vi "配置文件-查找多个键.vi"(6 "默认值":string[](array[string]), 8 "错误输入（无错误）":errorcluster, 9 "键名":string[](array[string]), 10 "章名":string, 11 "引用句柄输入":T1 caption="refnum") -> (0 "错误输出":errorcluster, 2 "查询结果":string[](array[string]), 3 "引用句柄输出":T1 caption="refnum out")   [LabVIEW 2014]
uses:
  <vilib>/Utility/config.llb/Config Data RefNum.ctl
  <vilib>/Utility/config.llb/Read Key (String).vi
  <vilib>/Utility/config.llb/NI_LVConfig.lvlib
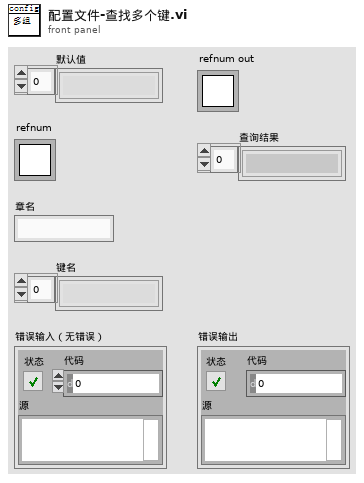
[diagram p1: front panel]
types:
  T1 = typedef "NI_LVConfig.lvlib/Config Data RefNum.ctl" = refnum<k1>
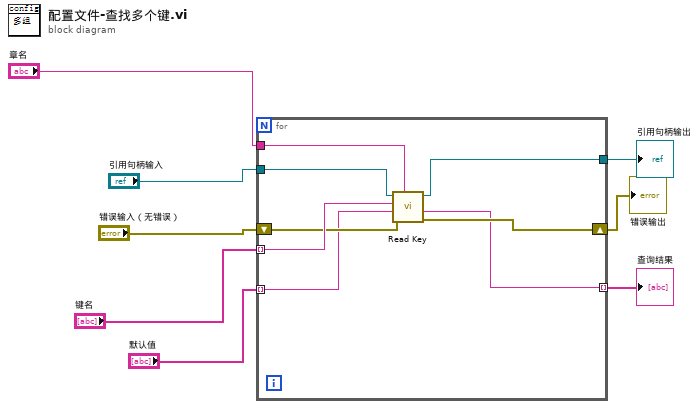
[diagram p0: block diagram]
diagram:
  n1 = for {
    tunnel: "默认值" -> [w9] mode=indexing
    tunnel: "键名" -> [w14] mode=indexing
    tunnel: "引用句柄输入" -> [w16]
    tunnel: "章名" -> [w15]
    shift-right: [w12] -> w6
    shift-left: "错误输入（无错误）" -> [w13]
    tunnel: [w11] -> w7
    tunnel: [w10] -> w8 mode=indexing
    n2 = call-poly <vilib>:"Read Key.vi"("section"=w15, "error in (no error)"=w13, "default value"=w9, "key"=w14, "refnum"=w16) -> ("error out"=w12:errorcluster, "value"=w10:string, "refnum out"=w11:T1)  [unwired: 3 in, 1 out]
  }
  "查询结果" <- w8
  "引用句柄输出" <- w7
  "错误输出" <- w6
